vi "Length_5_R1.vi"() -> ()   [LabVIEW 2020]
uses:
  Support/Controls/Clst_Initialize Input.ctl
  Support/Controls/Clst_Result inspec.ctl
  Support/Controls/Cmd_Var Data IO.ctl
  Support/Controls/Cmd_Mouse Popup.ctl
  Variables/Global_Cal Info.vi
panel:
  out "기준기선택":string
  in  "Measured 2":string[][](table)
  in  "Measured_ADJ":string[][](table) caption="조정후"
  out "최소범위":string
  in  "표시방식":string(combo)
  out "단위":string
  out "최대범위":string
  in  "Spec 변경":bool
  in  "Random":bool
  out "Resolution":string[][](table) caption="Spec"
  out "Spec":string[][](table)
  out "제목":string
  out "에러 출력":errorcluster
  out "Condition":string[][](table) caption="2. 직선성 시험"
  in  "최소눈금":string(combo)
  in  "Measured":string[][](table) caption="조정전"
  out "Load?":bool
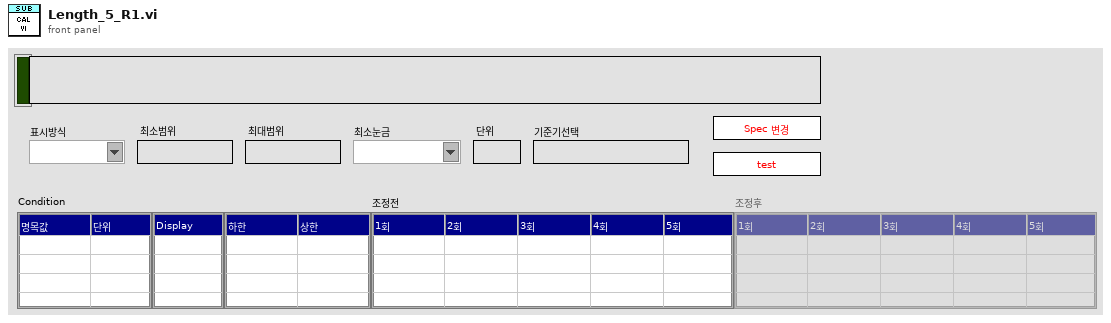
[diagram p1: front panel]
types:
  T1 = typedef "Cmd_Mouse Popup.ctl" = enum16{"활성화", "메뉴선택"}
  T2 = cluster{"Shift":bool, "Ctrl":bool, "Alt":bool, "Cmd":bool, "Opt":bool}
  T3 = typedef "Clst_Initialize Input.ctl" = cluster{"Initialize 1":cluster{"Condition":refnum<vi>[], "Spec":refnum<vi>[], "Measured":refnum<vi>[], "Resolution":refnum<vi>[], "Func_ext":string, "제목":refnum<vi>, "Measured_ADJ":refnum<vi>[]}, "Initialize 2":cluster{"문자열":refnum<vi>[], "콤보박스":refnum<vi>[], "링":refnum<vi>[], "열거형":refnum<vi>[], "테이블":refnum<vi>[], "여러열":refnum<vi>[], "디지털(DBL)":refnum<vi>[], "3D string":refnum<vi>[], "ctrl":refnum<vi>[], "boolean":refnum<vi>[]}}
  T4 = typedef "Clst_Result inspec.ctl" = cluster{"분해능":string, "문자열 1":string, "문자열 2":string, "숫자형 1":i32, "숫자형 2":i32, "숫자형 3":dbl, "문자배열 1D":string[], "문자배열 2D":string[][], "문자배열 3D":string[][][], "문자배열 4D":string[][][][], "불리언 1D":bool[]}
  T5 = typedef "Cmd_Var Data IO.ctl" = enum16{"Condition", "Condition Default", "Condition_Temp", "Resolution", "Resolution Default", "Resolution Old", "Spec", "Spec Default", "Spec Old", "Spec Temp", "Result", "Result2", "Result3", "Result_Temp", "Result_ADJ", "Result_ADJ2", "STD1", "STD2", "STD3", "STD4", "STD5", "STD Temp", "CMC", "CMC Default"}
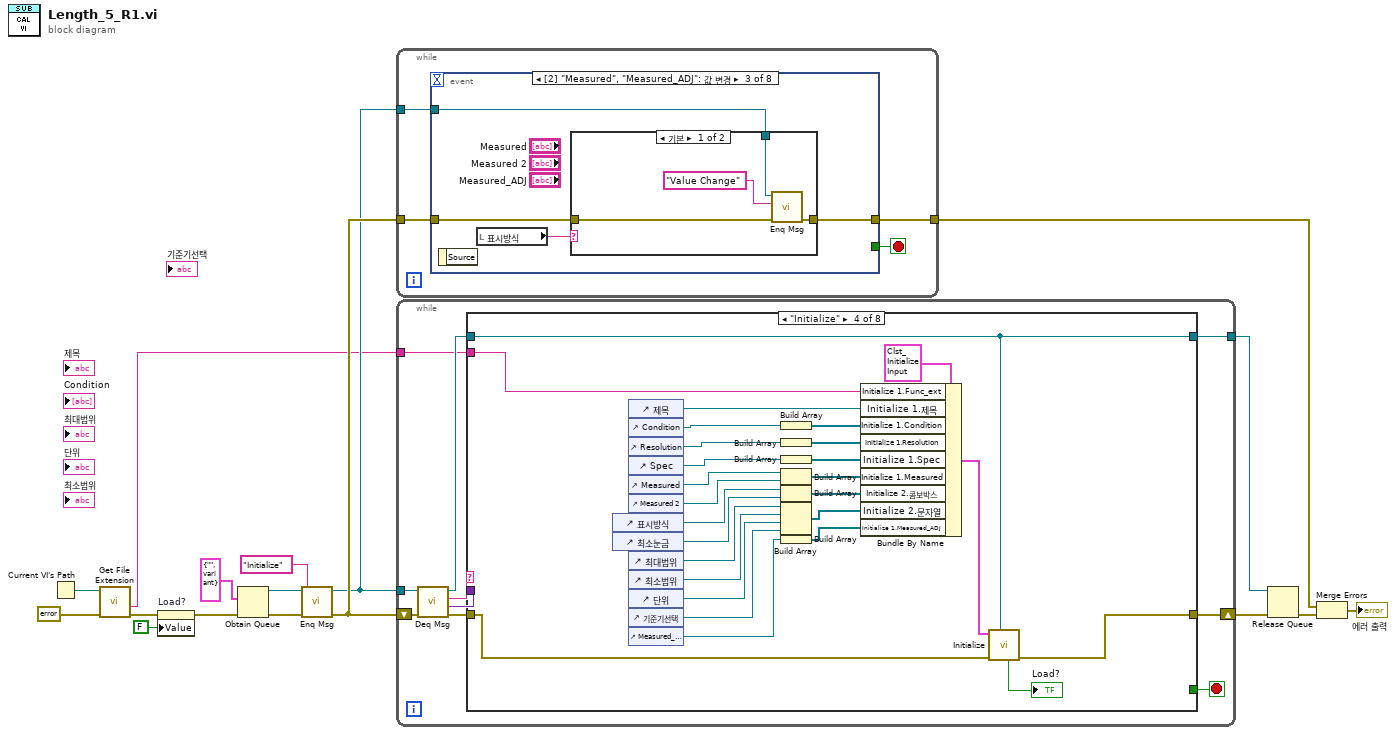
[diagram p0: block diagram]
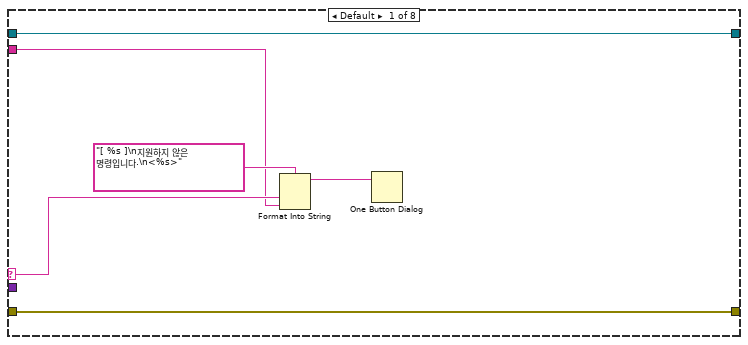
[diagram p2: hidden frame]
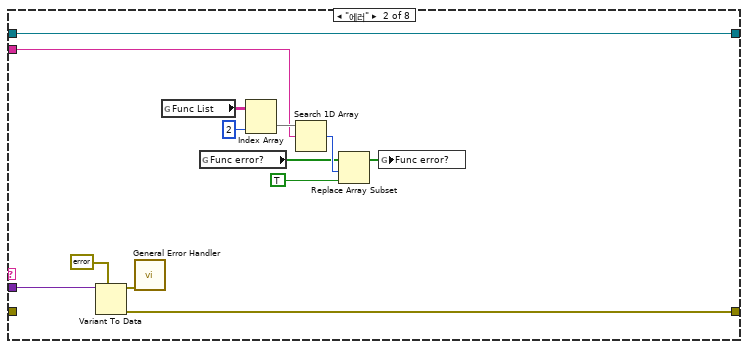
[diagram p3: hidden frame]
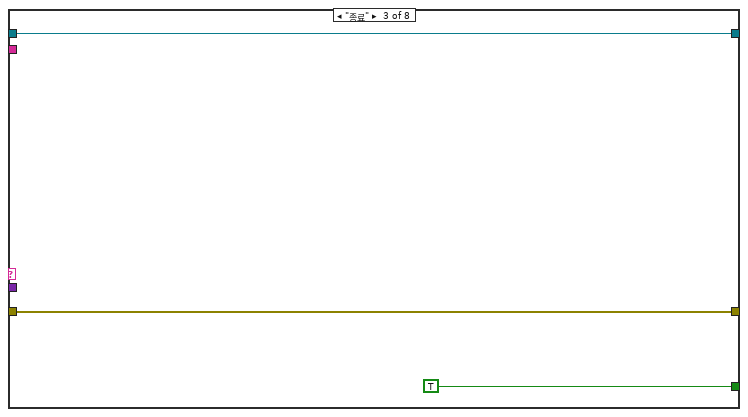
[diagram p4: hidden frame]
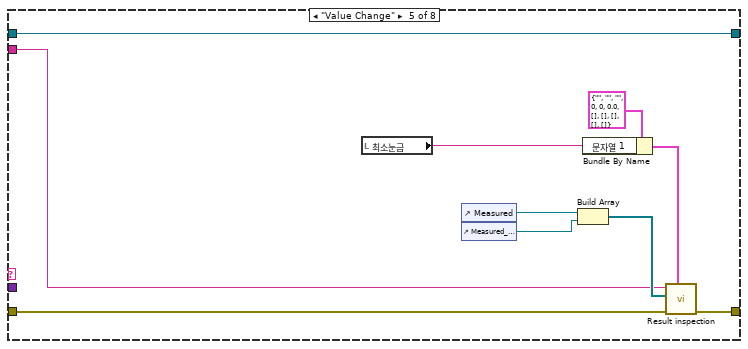
[diagram p5: hidden frame]
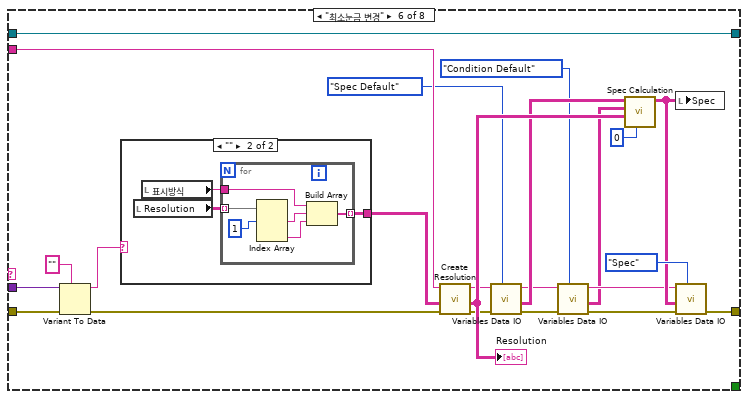
[diagram p6: hidden frame]
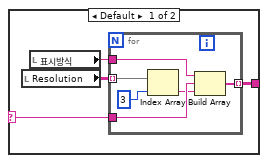
[diagram p7: hidden frame]
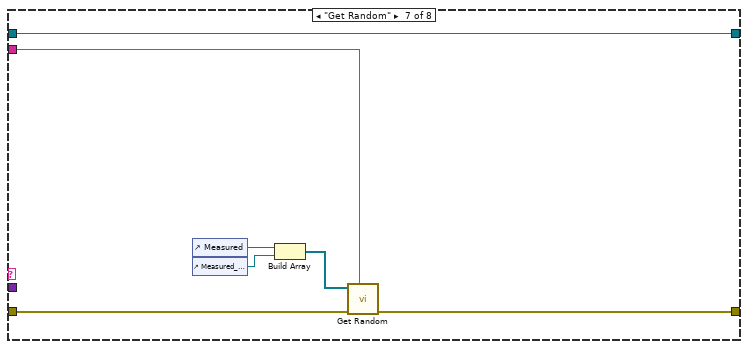
[diagram p8: hidden frame]
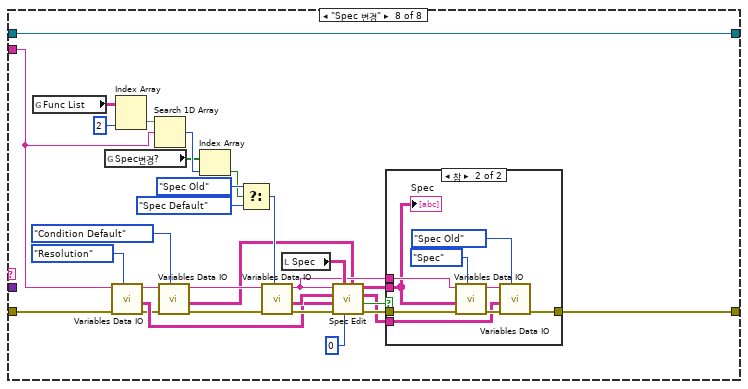
[diagram p9: hidden frame]
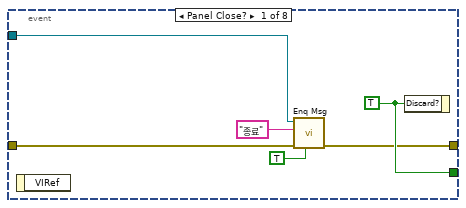
[diagram p11: hidden frame]
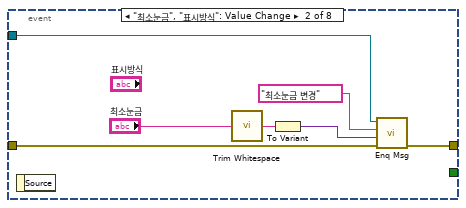
[diagram p12: hidden frame]
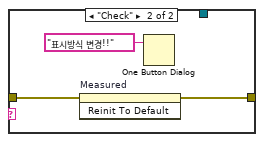
[diagram p13: hidden frame]
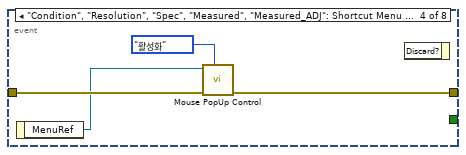
[diagram p14: hidden frame]
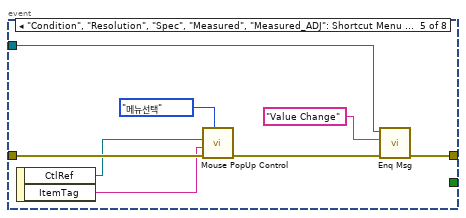
[diagram p15: hidden frame]
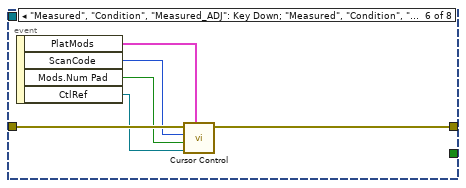
[diagram p16: hidden frame]
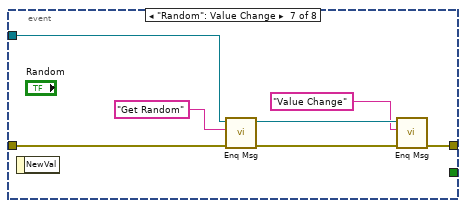
[diagram p17: hidden frame]
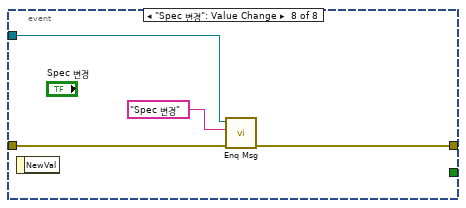
[diagram p18: hidden frame]
diagram:
  n1 = Current VI's Path() -> (path=w5:path)
  n2 = call <vilib>:"Get File Extension.vi"("error in (no error)"=errorcluster {"status"=FALSE, "code"=0, "source"=""} ("에러 상수"), "file"=w5) -> ("error out"=w3:errorcluster, "filename without extension"=w4:string)  [unwired: 5 in, 3 out]
  n3 = property on="Load?" class="Bool (엄격한)"(error in=w3, "Value"=FALSE ("Load?")) -> (error out=w2:errorcluster)  [unwired: 1 in, 1 out]
  n4 = Obtain Queue(element data type=cluster{"메세지":string, "값":variant} {"메세지"="", "값"=variant} ("Message Cluster"), error in (no error)=w2) -> (queue out=w14:refnum<queue>, error out=w16:errorcluster)  [unwired: 3 in, 1 out]
  n5 = call "Enq Msg.vi"("에러 입력(에러 없음)"=w16, "메세지"="Initialize", "큐 입력"=w14) -> ("에러 출력"=w15:errorcluster, "큐 출력"=w12:refnum<queue>)  [unwired: 7 in]
  n6 = while {
    tunnel: w15 -> [w19]
    tunnel: w12 -> [w20]
    tunnel: [w18] -> w9
    stop <- w21 stop-if-true
    n7 = event shown="[2] \"Measured\", \"Measured_ADJ\": 값 변경" {
      selector: _ -> [_ _ _ _ _ _ _ _]
      dyn-events: _ -> [_ _ _ _ _ _ _ _]
      timeout: _ -> [_ _ _ _ _ _ _ _]
      tunnel: [w27 _ _ _ _ _ _ _] -> w21
      tunnel: w20 -> [w25 w33 w38 _ w50 _ w68 w72]
      tunnel: w19 -> [w26 w34 w36 w49 w57 w63 w69 w73]
      tunnel: [w23 w32 w37 w48 w51 w62 w64 w71] -> w18
      event Panel Close? {
        w27 = TRUE ("버림?")
        n8 = event-data() -> ()  [unwired: 1 in, 1 out]
        n9 = call "Enq Msg.vi"("우선순위 메시지?"=TRUE, "에러 입력(에러 없음)"=w26, "메세지"="종료", "큐 입력"=w25) -> ("에러 출력"=w23:errorcluster)  [unwired: 6 in, 1 out]
        n10 = event-data("Discard?"=w27) -> ()  [unwired: 1 in, 1 out]
      }
      event "최소눈금", "표시방식": Value Change {
        n11 = event-data() -> ()  [unwired: 1 in, 1 out]
        n12 = call <vilib>:"Trim Whitespace.vi"("string"="최소눈금") -> ("trimmed string"=w30:string)  [unwired: 1 in]
        n13 = To Variant(anything=w30) -> (Variant=w28:variant)
        n14 = call "Enq Msg.vi"("에러 입력(에러 없음)"=w34, "값"=w28, "메세지"="최소눈금 변경", "큐 입력"=w33) -> ("에러 출력"=w32:errorcluster)  [unwired: 6 in, 1 out]
      }
      event "Measured", "Measured_ADJ": Value Change {
        n15 = event-data() -> ()  [unwired: 1 in, 1 out]
        n16 = local read "표시방식"() -> (w35:string)
        n17 = case shown="기본" w35 {
          tunnel: w38 -> [w42 _]
          tunnel: [w41 w43] -> w37
          tunnel: w36 -> [w40 w44]
          frame Default {
            n18 = call "Enq Msg.vi"("에러 입력(에러 없음)"=w40, "메세지"="Value Change", "큐 입력"=w42) -> ("에러 출력"=w41:errorcluster)  [unwired: 7 in, 1 out]
          }
          frame "Check" {
            n19 = invoke on="Measured" class="Tbl (엄격한)" method="Reinit To Default"(error in=w44) -> (error out=w43:errorcluster)  [unwired: 2 in, 2 out]
            n20 = One Button Dialog(message="표시방식 변경!!" ("메시지")) -> ()  [unwired: 1 in, 1 out]
          }
        }
      }
      event "Condition", "Resolution", "Spec", "Measured", "Measured_ADJ": Shortcut Menu Activation? {
        n21 = event-data() -> ("MenuRef"=w47:refnum<k9>)  [unwired: 1 in]
        n22 = call "Mouse PopUp Control.vi"("type"=Cmd_Mouse_Popup."활성화", "error in"=w49, "메뉴 참조"=w47) -> ("error out"=w48:errorcluster)  [unwired: 8 in]
        n23 = event-data() -> ()  [unwired: 2 in, 1 out]
      }
      event "Condition", "Resolution", "Spec", "Measured", "Measured_ADJ": Shortcut Menu Selection (User) {
        n24 = event-data() -> ("CtlRef"=w55:refnum<vi>, "ItemTag"=w54:string)  [unwired: 1 in]
        n25 = call "Mouse PopUp Control.vi"("type"=Cmd_Mouse_Popup."메뉴선택", "error in"=w57, "아이템 태그"=w54, "Tbl 참조 번호"=w55) -> ("error out"=w52:errorcluster)  [unwired: 7 in]
        n26 = call "Enq Msg.vi"("에러 입력(에러 없음)"=w52, "메세지"="Value Change", "큐 입력"=w50) -> ("에러 출력"=w51:errorcluster)  [unwired: 7 in, 1 out]
      }
      event "Measured", "Condition", "Measured_ADJ": Key Down; "Measured", "Condition", "Measured_ADJ": Key Repeat {
        n27 = event-data() -> ("PlatMods"=w58:T2, "ScanCode"=w61:i16, "Mods.Num Pad"=w60:bool, "CtlRef"=w59:refnum<vi>)  [unwired: 1 in]
        n28 = call "Cursor Control.vi"("플랫폼 조합키"=w58, "참조"=w59, "Num Pad"=w60, "ScanCode"=w61, "error in"=w63) -> ("error out"=w62:errorcluster)  [unwired: 5 in, 1 out]
      }
      event "Random": Value Change {
        n29 = event-data() -> ()  [unwired: 1 in, 1 out]
        n30 = call "Enq Msg.vi"("에러 입력(에러 없음)"=w69, "메세지"="Get Random", "큐 입력"=w68) -> ("에러 출력"=w67:errorcluster, "큐 출력"=w66:refnum<queue>)  [unwired: 7 in]
        n31 = call "Enq Msg.vi"("에러 입력(에러 없음)"=w67, "메세지"="Value Change", "큐 입력"=w66) -> ("에러 출력"=w64:errorcluster)  [unwired: 7 in, 1 out]
      }
      event "Spec 변경": Value Change {
        n32 = event-data() -> ()  [unwired: 1 in, 1 out]
        n33 = call "Enq Msg.vi"("에러 입력(에러 없음)"=w73, "메세지"="Spec 변경", "큐 입력"=w72) -> ("에러 출력"=w71:errorcluster)  [unwired: 7 in, 1 out]
      }
    }
  }
  n34 = while {
    shift-right: [w84] -> w11
    shift-left: w15 -> [w83]
    tunnel: w12 -> [w81]
    tunnel: [w76] -> w10
    tunnel: w4 -> [w75]
    stop <- w77 stop-if-true
    n35 = call "Deq Msg.vi"("에러 입력(에러 없음)"=w83, "큐 입력"=w81) -> ("에러 출력"=w82:errorcluster, "값"=w78:variant, "메세지"=w80:string, "큐 출력"=w79:refnum<queue>)  [unwired: 6 in]
    n36 = case shown="\"Initialize\"" w80 {
      selector: w80 -> [w86 _ _ _ _ _ _ _]
      tunnel: w82 -> [w90 _ w106 w133 w137 w165 w188 w215]
      tunnel: [w90 w100 w106 w123 w142 w158 w189 w218] -> w84
      tunnel: w79 -> [w89 w99 w104 w117 w143 w166 w192 w222]
      tunnel: w78 -> [_ w101 _ _ _ w164 _ _]
      tunnel: [_ _ TRUE ("버림?") _ _ _ _ _] -> w77
      tunnel: [w89 w99 w104 w117 w143 w166 w192 w222] -> w76
      tunnel: w75 -> [w85 w91 _ w118 w136 w162 w187 w200]
      frame Default {
        n37 = Format Into String(format string="[ %s ]\n지원하지 않은 명령입니다.\n<%s>" ("메시지"), w86, w85) -> (resulting string=w87:string)  [unwired: 2 in, 1 out]
        n38 = One Button Dialog(message=w87) -> ()  [unwired: 1 in, 1 out]
      }
      frame "에러" {
        n39 = Variant To Data(type=errorcluster {"status"=FALSE, "code"=0, "source"=""} ("에러 출력"), Variant=w101) -> (data=w103:errorcluster, error out=w100:errorcluster)  [unwired: 1 in]
        n40 = call <vilib>:"General Error Handler.vi"("error in (no error)"=w103) -> ()  [unwired: 10 in, 5 out]
        n41 = global read "Global_Cal Info.vi" "Func List"() -> (w93:string[][])
        n42 = global read "Global_Cal Info.vi" "Func error?"() -> (w96:bool[])
        n43 = Index Array(array=w93, index (col)=2 ("비활성화된 인덱스 (열)")) -> (element=w94:string[])  [unwired: 1 in]
        n44 = Search 1D Array(1D array=w94, element=w91) -> (index of element=w97:i32)  [unwired: 1 in]
        n45 = Replace Array Subset(array=w96, new element=TRUE ("새 원소/부분배열"), index=w97) -> (w98:bool[])
        n46 = global write "Global_Cal Info.vi" "Func error?"(w98) -> ()
      }
      frame "종료" {
      }
      frame "Initialize" {
        n47 = control-ref of="표시방식"() -> (w116:refnum<vi>)
        n48 = control-ref of="최소눈금"() -> (w126:refnum<vi>)
        n49 = control-ref of="제목"() -> (w124:refnum<vi>)
        n50 = control-ref of="Condition"() -> (w130:refnum<vi>)
        n51 = control-ref of="Resolution"() -> (w119:refnum<vi>)
        n52 = control-ref of="Spec"() -> (w122:refnum<vi>)
        n53 = control-ref of="Measured"() -> (w127:refnum<vi>)
        n54 = control-ref of="Measured 2"() -> (w108:refnum<vi>)
        n55 = control-ref of="최대범위"() -> (w112:refnum<vi>)
        n56 = control-ref of="최소범위"() -> (w113:refnum<vi>)
        n57 = control-ref of="단위"() -> (w115:refnum<vi>)
        n58 = control-ref of="기준기선택"() -> (w107:refnum<vi>)
        n59 = control-ref of="Measured_ADJ"() -> (w110:refnum<vi>)
        n60 = Build Array(w130) -> (w129:refnum<vi>[])
        n61 = Build Array(w119) -> (w120:refnum<vi>[])
        n62 = Build Array(w122) -> (w121:refnum<vi>[])
        n63 = Build Array(w127, w108) -> (w128:refnum<vi>[])
        n64 = Build Array(w116, w126) -> (w125:refnum<vi>[])
        n65 = Build Array(w112, w113, w115, w107) -> (w114:refnum<vi>[])
        n66 = Build Array(w110) -> (w109:refnum<vi>[])
        n67 = Bundle By Name(cluster=T3 {"Initialize 1"={"Condition"=[], "Spec"=[], "Measured"=[], "Resolution"=[], "Func_ext"="", "제목"=refnum, "Measured_ADJ"=[]}, "Initialize 2"={"문자열"=[], "콤보박스"=[], "링"=[], "열거형"=[], "테이블"=[], "여러열"=[], "디지털(DBL)"=[], "3D string"=[], "ctrl"=[], "boolean"=[]}} ("입력 클러스터"), "Initialize 1.Func_ext"=w118, "Initialize 1.제목"=w124, "Initialize 1.Condition"=w129, "Initialize 1.Resolution"=w120, "Initialize 1.Spec"=w121, "Initialize 1.Measured"=w128, "Initialize 2.콤보박스"=w125, "Initialize 2.문자열"=w114, "Initialize 1.Measured_ADJ"=w109) -> (w131:T3)
        n68 = call "Initialize.vi"("큐 입력"=w117, "error in"=w133, "입력 클러스터"=w131) -> ("error out"=w123:errorcluster, "Load?"=→"Load?":bool)  [unwired: 5 in, 2 out]
      }
      frame "Value Change" {
        n69 = local read "최소눈금"() -> (w135:string)
        n70 = control-ref of="Measured"() -> (w141:refnum<vi>)
        n71 = control-ref of="Measured_ADJ"() -> (w134:refnum<vi>)
        n72 = Build Array(w141, w134) -> (w140:refnum<vi>[])
        n73 = Bundle By Name(cluster=T4 {"분해능"="", "문자열 1"="", "문자열 2"="", "숫자형 1"=0, "숫자형 2"=0, "숫자형 3"=0.0, "문자배열 1D"=[], "문자배열 2D"=[], "문자배열 3D"=[], "문자배열 4D"=[], "불리언 1D"=[]} ("입력 클러스터"), "문자열 1"=w135) -> (w138:T4)
        n74 = call "Result inspection.vi"("입력 클러스터"=w138, "error in"=w137, "Ref. Data (Inspection)"=w140, "Func ext"=w136) -> ("error out"=w142:errorcluster)  [unwired: 4 in, 3 out]
      }
      frame "최소눈금 변경" {
        n75 = Variant To Data(error in=w165, type="", Variant=w164) -> (data=w151:string, error out=w153:errorcluster)
        n76 = case shown="\"\"" w151 {
          selector: w151 -> [w167 _]
          tunnel: [w170 w179] -> w152
          frame Default {
            n77 = local read "Resolution"() -> (w169:string[][])
            n78 = local read "표시방식"() -> (w168:string)
            n79 = for {
              tunnel: w169 -> [w176] mode=indexing
              tunnel: w167 -> [w175]
              tunnel: [w173] -> w170 mode=indexing
              tunnel: w168 -> [w172]
              n80 = Index Array(array=w176, index=3 ("인덱스")) -> (element=w174:string)
              n81 = Build Array(w172, w175, w174) -> (w173:string[])
            }
          }
          frame "" {
            n82 = local read "Resolution"() -> (w178:string[][])
            n83 = local read "표시방식"() -> (w177:string)
            n84 = for {
              tunnel: w178 -> [w185] mode=indexing
              tunnel: [w184] -> w179 mode=indexing
              tunnel: w177 -> [w183]
              n85 = Index Array(array=w185, index #1=1 ("인덱스")) -> (element #1=w181:string, element #3=w180:string)  [unwired: 2 in, 1 out]
              n86 = Build Array(w183, w181, w180) -> (w184:string[])
            }
          }
        }
        n87 = call "Create Resolution.vi"("에러 입력(에러 없음)"=w153, "Resolution"=w152, "Func_ext"=w162) -> ("에러 출력"=w156:errorcluster, "Resolution Out"=w159:string[][], "Func_ext 출력"=w155:string)  [unwired: 6 in]
        "Resolution" <- w159
        n88 = call "Variables Data IO.vi"("Select"=Cmd_Var_Data_IO."Spec Default", "error in"=w156, "Func_ext"=w155) -> ("error out"=w147:errorcluster, "Data Out"=w154:string[][], "Func_ext Out"=w148:string)  [unwired: 6 in]
        n89 = call "Variables Data IO.vi"("Select"=Cmd_Var_Data_IO."Condition Default", "error in"=w147, "Func_ext"=w148) -> ("error out"=w145:errorcluster, "Data Out"=w144:string[][], "Func_ext Out"=w146:string)  [unwired: 6 in]
        n90 = call "Spec Calculation.vi"("기준값 열번호"=0 ("열번호(기준값)"), "Resolution"=w159, "Condition in"=w144, "Spec Default"=w154) -> ("Spec out"=w150:string[][])  [unwired: 6 in, 1 out]
        n91 = local write "Spec"(w150) -> ()
        n92 = call "Variables Data IO.vi"("Select"=Cmd_Var_Data_IO."Spec", "error in"=w145, "Data In"=w150, "Func_ext"=w146) -> ("error out"=w158:errorcluster)  [unwired: 5 in, 2 out]
      }
      frame "Get Random" {
        n93 = control-ref of="Measured"() -> (w191:refnum<vi>)
        n94 = control-ref of="Measured_ADJ"() -> (w186:refnum<vi>)
        n95 = Build Array(w191, w186) -> (w190:refnum<vi>[])
        n96 = call "Get Random.vi"("Func_Ext"=w187, "에러 입력"=w188, "Meas"=w190) -> ("에러 출력"=w189:errorcluster)  [unwired: 7 in, 1 out]
      }
      frame "Spec 변경" {
        n97 = global read "Global_Cal Info.vi" "Func List"() -> (w205:string[][])
        n98 = global read "Global_Cal Info.vi" "Spec변경?"() -> (w201:bool[])
        n99 = call "Variables Data IO.vi"("Select"=Cmd_Var_Data_IO."Resolution", "error in"=w215, "Func_ext"=w200) -> ("error out"=w198:errorcluster, "Data Out"=w209:string[][], "Func_ext Out"=w196:string)  [unwired: 6 in]
        n100 = Index Array(array=w205, index (col)=2 ("비활성화된 인덱스 (열)")) -> (element=w203:string[])  [unwired: 1 in]
        n101 = Search 1D Array(1D array=w203, element=w200) -> (index of element=w202:i32)  [unwired: 1 in]
        n102 = call "Variables Data IO.vi"("Select"=Cmd_Var_Data_IO."Condition Default", "error in"=w198, "Func_ext"=w196) -> ("error out"=w197:errorcluster, "Data Out"=w193:string[][], "Func_ext Out"=w195:string)  [unwired: 6 in]
        n103 = Index Array(array=w201, index=w202) -> (element=w206:bool)
        n104 = Select(t=Cmd_Var_Data_IO."Spec Old" ("Select"), s=w206, f=Cmd_Var_Data_IO."Spec Default" ("Select")) -> (s? t:f=w199:T5)
        n105 = call "Variables Data IO.vi"("Select"=w199, "error in"=w197, "Func_ext"=w195) -> ("error out"=w217:errorcluster, "Data Out"=w210:string[][], "Func_ext Out"=w211:string)  [unwired: 6 in]
        n106 = local read "Spec"() -> (w212:string[][])
        n107 = call "Spec Edit.vi"("Condition"=w193, "열번호(기준값)"=0, "Spec Value"=w212, "에러 입력(에러 없음)"=w217, "Resolution"=w209, "Spec Default"=w210, "Func_ext"=w211) -> ("에러 출력"=w219:errorcluster, "변경?"=w220:bool, "Spec Default out"=w214:string[][], "Spec 출력"=w221:string[][])  [unwired: 1 in]
        n108 = case shown="참" w220 {
          tunnel: w221 -> [_ w229]
          tunnel: w219 -> [w223 w232]
          tunnel: [w223 w227] -> w218
          tunnel: w211 -> [_ w230]
          tunnel: w214 -> [_ w225]
          frame False {
          }
          frame True {
            n109 = call "Variables Data IO.vi"("Select"=Cmd_Var_Data_IO."Spec", "error in"=w232, "Data In"=w229, "Func_ext"=w230) -> ("error out"=w228:errorcluster, "Func_ext Out"=w226:string)  [unwired: 5 in, 1 out]
            n110 = call "Variables Data IO.vi"("Select"=Cmd_Var_Data_IO."Spec Old", "error in"=w228, "Data In"=w225, "Func_ext"=w226) -> ("error out"=w227:errorcluster)  [unwired: 5 in, 2 out]
            "Spec" <- w229
          }
        }
      }
    }
  }
  n111 = Release Queue(queue=w10, error in (no error)=w11) -> (error out=w8:errorcluster)  [unwired: 1 in, 2 out]
  n112 = Merge Errors(w9, w8) -> (→"에러 출력":errorcluster)
